vi "WPI_CameraStop.vi"(8 "error in (no error)":errorcluster, 11 "CameraDevRef":T1) -> (0 "error out":errorcluster, 3 "CameraDevRef":T1)   [LabVIEW 2017]
doc: "Stops acquiring image data from the camera you specify. If the count of acquisition requests is greater than one, this VI only decrements the number of acquisition requests by one.\n\nThis software is licensed. Open the labview\\readme\\WPI Robotics Library Open Source License.txt file for more information."
uses:
  <vilib>/Rock Robotics/WPI/Camera/WPI_CameraDevRef.ctl
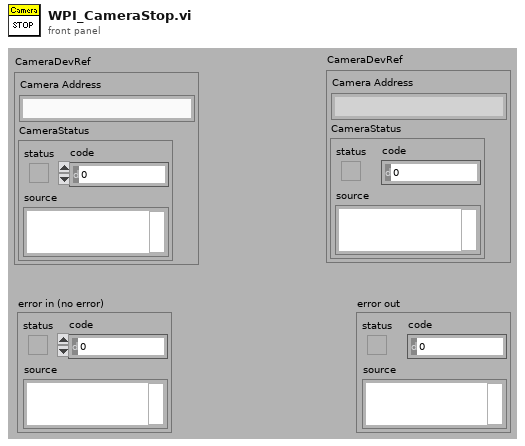
[diagram p1: front panel]
types:
  T1 = typedef "WPI_CameraDevRef.ctl" = cluster{"Camera Address":string, "CameraStatus":errorcluster}
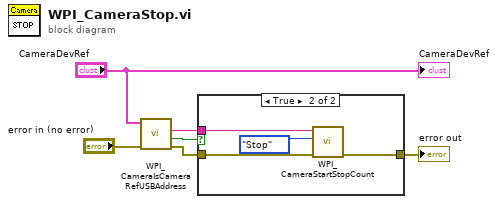
[diagram p0: block diagram]
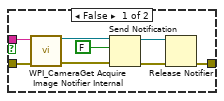
[diagram p2: hidden frame]
diagram:
  n1 = call <vilib>:"WPI_CameraIsCameraRefUSBAddress.vi"("error in (no error)"="error in (no error)", "CameraDevRef"="CameraDevRef") -> ("error out"=w2:errorcluster, "USB?"=w3:bool, "Camera Address Out"=w4:string)  [unwired: 6 in, 1 out]
  n2 = case shown="True" w3 {
    tunnel: [w12 w16] -> w6
    tunnel: w2 -> [w8 w17]
    tunnel: w4 -> [w7 w18]
    frame False {
      n3 = call <vilib>:"WPI_CameraGet Acquire Image Notifier Internal.vi"("error in (no error)"=w8, "Camera Address"=w7) -> ("error out"=w9:errorcluster, "Acquire Image Notifier"=w10:refnum<notifier>)  [unwired: 8 out]
      n4 = Send Notification(notification=FALSE, notifier=w10, error in (no error)=w9) -> (notifier out=w11:refnum<notifier>, error out=w13:errorcluster)
      n5 = Release Notifier(notifier=w11, error in (no error)=w13) -> (error out=w12:errorcluster)  [unwired: 3 out]
    }
    frame True {
      n6 = call <vilib>:"WPI_CameraStartStopCount.vi"("error in (no error)"=w17, "Action"=enum16{"Start", "Stop"}."Stop", "Camera Address Out"=w18) -> ("error out"=w16:errorcluster)  [unwired: 8 in]
    }
  }
  "error out" <- w6
  "CameraDevRef" <- "CameraDevRef"
